vi "MQTT_Q_ReadPublishedMessage.vi"(8 "error in (no error)":errorcluster, 10 "timeout ms (25000)":i32=25000, 11 "MQTT_Q In":refnum<class "MQTT_Q.lvclass">) -> (0 "error out":errorcluster, 1 "TimedOut":bool, 2 "Message":string, 3 "MQTT_Q Out":refnum<class "MQTT_Q.lvclass">, 5 "Topic":string)   [LabVIEW 2015, in "MQTT_Q.lvclass"]
uses:
  MQTT_Q.lvclass
  MQTT_Q_PVT_MessageType.ctl
panel:
  out "Message ID":u16=1 format="%x"
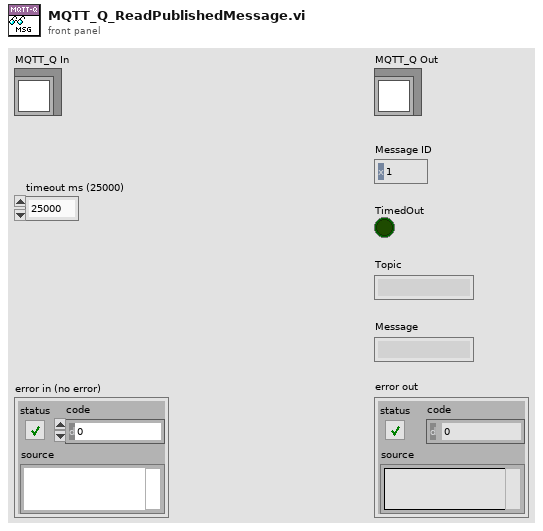
[diagram p1: front panel]
types:
  T1 = typedef "MQTT_Q.lvclass/MQTT_Q_PVT_MessageType.ctl" = enum32{"Reserved", "CONNECT", "CONNACK", "PUBLISH", "PUBACK", "PUBREC", "PUBREL", "PUBCOMP", "SUBSCRIBE", "SUBACK", "UNSUBSCRIBE", "UNSUBACK", "PINGREQ", "PINGRESP", "DISCONNECT", "Reserved2"}
  T2 = typedef "MQTT_Q.lvclass/MQTT_Q_PVT_FixedHeader.ctl" = cluster{"MessageType":T1, "DUP Flag":bool, "QoS Level":T3, "RETAIN":bool, "Remaining Length":u32}
  T3 = typedef "MQTT_Q.lvclass/MQTT_Q_QoS.ctl" = enum8{"At most once", "At least once", "Exactly once", "Reserved"}
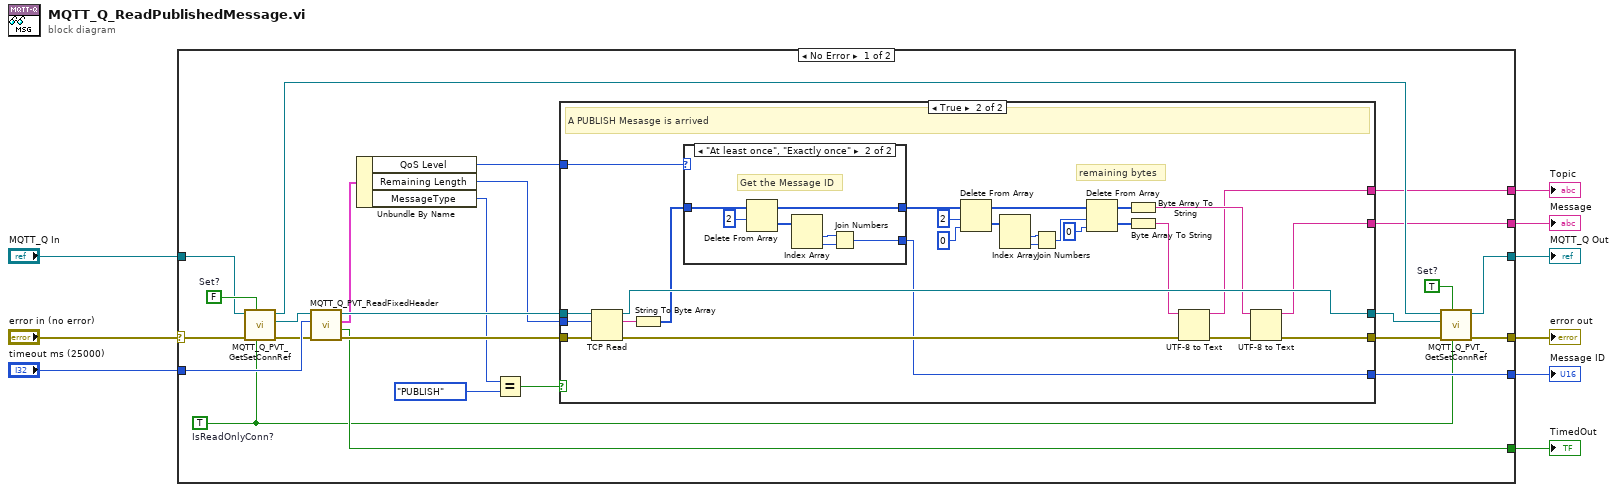
[diagram p0: block diagram]
diagram:
  n1 = case shown="No Error" "error in (no error)" {
    selector: "error in (no error)" -> [w31 w72]
    tunnel: [w17 w72] -> w8
    tunnel: "MQTT_Q In" -> [w29 w71]
    tunnel: [w34 w71] -> w6
    tunnel: "timeout ms (25000)" -> [w33 _]
    tunnel: [w11 _] -> w4
    tunnel: [w20 _] -> w3
    tunnel: [w19 _] -> w2
    tunnel: [w18 _] -> w1
    frame No Error {
      w10 = TRUE  # IsReadOnlyConn?
      w24 = TRUE  # Set?
      w32 = FALSE  # Set?
      n2 = call "MQTT_Q_PVT_GetSetConnRef.vi"("IsReadOnlyConn?"=w10, "Set?"=w32, "error in (no error)"=w31, "MQTT_Q in"=w29) -> ("error out"=w30:errorcluster, "connection ID Out"=w27:refnum<k5>, "MQTT_Q out"=w28:refnum<class "MQTT_Q.lvclass">)  [unwired: 5 in]
      n3 = call "MQTT_Q_PVT_ReadFixedHeader.vi"("error in"=w30, "timeout ms (25000)"=w33, "connection ID"=w27) -> ("error out"=w25:errorcluster, "TimedOut"=w11:bool, "Fixed Header"=w16:T2, "connection ID out"=w26:refnum<k5>)  [unwired: 5 in]
      n4 = Unbundle By Name(w16) -> ("QoS Level"=w13:T3, "Remaining Length"=w15:u32, "MessageType"=w14:T1)
      n5 = Equal?(x=w14, y=MQTT_Q_PVT_MessageType."PUBLISH") -> (x = y?=w21:bool)
      n6 = case shown="True" w21 {
        tunnel: w15 -> [_ w62]
        tunnel: w26 -> [w35 w61]
        tunnel: w25 -> [w36 w60]
        tunnel: w13 -> [_ w40]
        tunnel: [w35 w58] -> w22
        tunnel: [w36 w56] -> w23
        tunnel: [_ w55] -> w20
        tunnel: [_ w37] -> w19
        tunnel: [_ w39] -> w18
        frame False {
          # "Not a PUBLISH message...."
        }
        frame True {
          # "remaining bytes"
          # "A PUBLISH Mesasge is arrived"
          n7 = TCP Read(connection ID=w61, bytes to read=w62, error in (no error)=w60) -> (connection ID out=w58:refnum<k5>, data out=w59:string, error out=w43:errorcluster)  [unwired: 2 in]
          n8 = String To Byte Array(string=w59) -> (unsigned byte array=w41:u8[])
          n9 = case shown="\"At least once\", \"Exactly once\"" w40 {
            tunnel: w41 -> [w63 w70]
            tunnel: [w63 w65] -> w54
            tunnel: [_ w64] -> w37
            frame "At most once", Default {
            }
            frame "At least once", "Exactly once" {
              # "Get the Message ID"
              n10 = Delete From Array(array=w70, length=2) -> (deleted portion=w68:u8[], array with subset deleted=w65:u8[])  [unwired: 1 in]
              n11 = Index Array(array=w68) -> (element #1=w66:u8, element #2=w67:u8)  [unwired: 2 in]
              n12 = Join Numbers(hi=w66, lo=w67) -> ((hi.lo)=w64:u16)
            }
          }
          n13 = Delete From Array(array=w54, length=2, index=0) -> (deleted portion=w51:u8[], array with subset deleted=w50:u8[])
          n14 = Index Array(array=w51) -> (element #1=w48:u8, element #2=w49:u8)  [unwired: 2 in]
          n15 = Join Numbers(hi=w48, lo=w49) -> ((hi.lo)=w45:u16)
          n16 = Delete From Array(array=w50, length=w45, index=0) -> (deleted portion=w52:u8[], array with subset deleted=w38:u8[])
          n17 = Byte Array To String(unsigned byte array=w38) -> (string=w57:string)
          n18 = Byte Array To String(unsigned byte array=w52) -> (string=w44:string)
          n19 = UTF-8 to Text(8:w43, 11:w44) -> (0:w42:errorcluster, 3:w39:string)  [unwired: 1 in]
          n20 = UTF-8 to Text(8:w42, 11:w57) -> (0:w56:errorcluster, 3:w55:string)  [unwired: 1 in]
        }
      }
      n21 = call "MQTT_Q_PVT_GetSetConnRef.vi"("IsReadOnlyConn?"=w10, "Set?"=w24, "error in (no error)"=w23, "connection ID In"=w22, "MQTT_Q in"=w28) -> ("error out"=w17:errorcluster, "MQTT_Q out"=w34:refnum<class "MQTT_Q.lvclass">)  [unwired: 4 in, 1 out]
    }
    frame Error {
    }
  }
  "error out" <- w8
  "MQTT_Q Out" <- w6
  "TimedOut" <- w4
  "Message" <- w3
  "Topic" <- w1
  "Message ID" <- w2
